vi "Climb.vi"(11 "Buttons":bool[](array[boolean])) -> ()   [LabVIEW 2015]
uses:
  Utilities/ReadyClimber.ctl
  Utilities/Climb.ctl
  Utilities/GeneralGlobals.vi
  Utilities/MotorPositionGlobals.vi
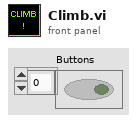
[diagram p1: front panel]
types:
  T1 = typedef "Climb.ctl" = enum16{"WaitingForInput", "ArmUp", "CloseServo", "Climb"}
  T2 = typedef "ReadyClimber.ctl" = enum16{"WaitingForInput", "ArmUp", "OpenServo", "LiftUp"}
  T3 = typedef "WPI_MotorControlDeviceRef.ctl" = cluster{"DeviceStatus":errorcluster, "Type":T4, "PWM":cluster{"PWM Channel":T5, "DeadBand":T6}, "CAN":cluster{"Device Number":u8, "Control Mode":T7, "Semaphore":T8, "Max Vout":dbl, "TalonSRX Control Mode":T9}, "Invert":bool}
  T4 = typedef "WPI_MotorControlType.ctl" = enum16{"PWM", "CAN", "CANTalonSRX"}
  T5 = typedef "FPGA_DIOPWMChannel.ctl" = enum8{"PWM 0", "PWM 1", "PWM 2", "PWM 3", "PWM 4", "PWM 5", "PWM 6", "PWM 7", "PWM 8", "PWM 9", "PWM MXP 0", "PWM MXP 1", "PWM MXP 2", "PWM MXP 3", "PWM MXP 4", "PWM MXP 5", "PWM MXP 6", "PWM MXP 7", "PWM MXP 8", "PWM MXP 9", "Invalid"}
  T6 = typedef "WPI_PWMDeadband.ctl" = cluster{"Name":string, "maxPositivePwm":i32, "minPositivePwm":i32, "centerPwm":i32, "maxNegativePwm":i32, "minNegativePwm":i32, "angularRange":u16}
  T7 = typedef "WPI_CANJaguar_ControlMode.ctl" = enum8{"Percent VBus", "Current", "Speed", "Position", "Voltage"}
  T8 = typedef "Semaphore RefNum" = refnum<k1>
  T9 = typedef "WPI_CANTalonSRX_APIControlMode.ctl" = enum8{"Percent VBus", "Speed", "Position", "Slave", "Unchanged / Invalid", "Voltage Compensation", "Current", "Motion Profile"}
  T10 = typedef "WPI_ServoDeviceRef.ctl" = cluster{"DeviceStatus":errorcluster, "PWM Channel":T5, "DeadBand":T6}
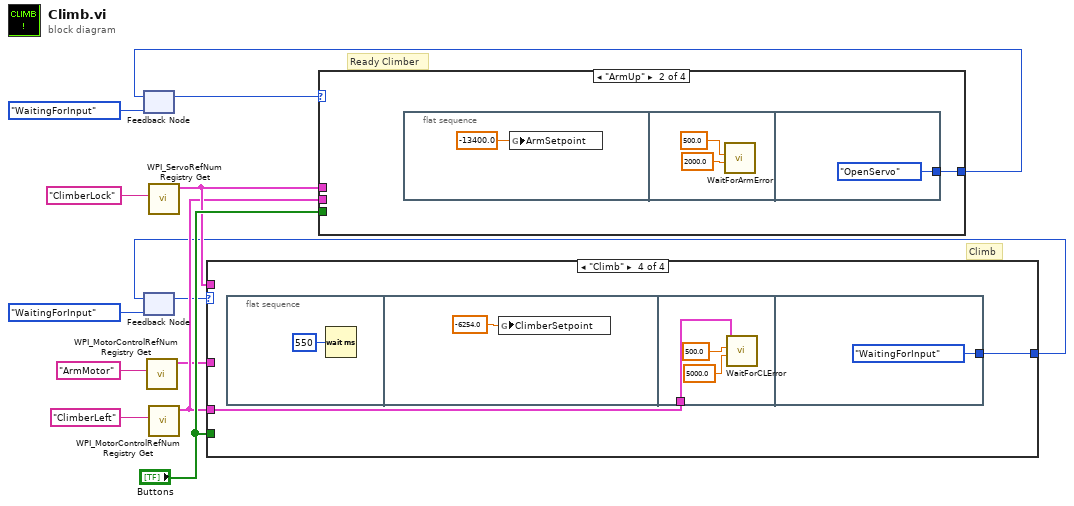
[diagram p0: block diagram]
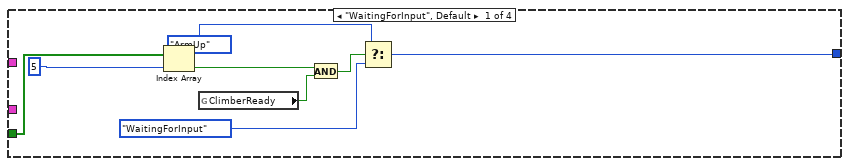
[diagram p2: hidden frame]
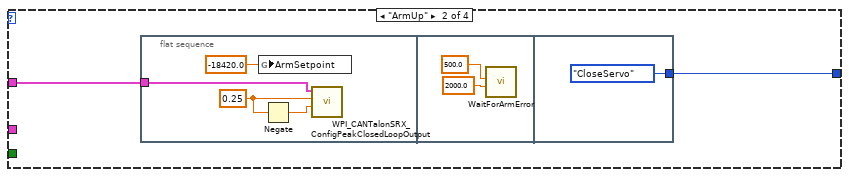
[diagram p3: hidden frame]
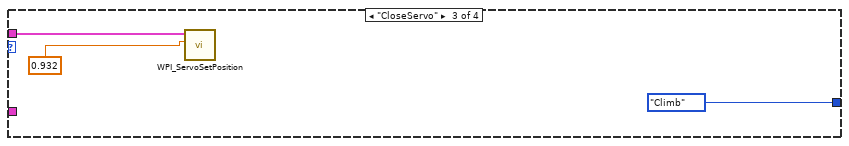
[diagram p4: hidden frame]
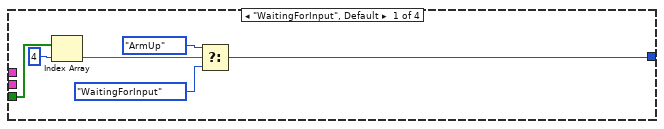
[diagram p5: hidden frame]
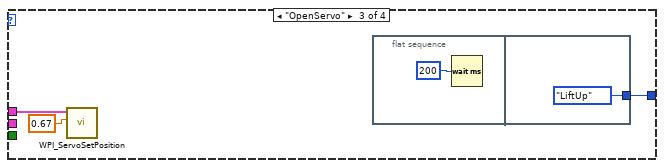
[diagram p6: hidden frame]
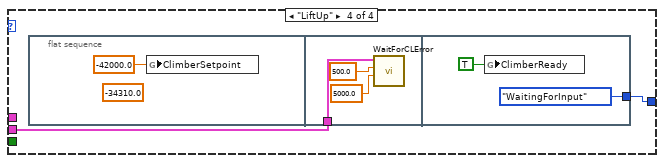
[diagram p7: hidden frame]
diagram:
  # "Climb"
  # "Ready Climber"
  n1 = feedback #1(ReadyClimber."WaitingForInput" ("Enum")) -> (w10:T2)
  n2 = feedback #2(Climb."WaitingForInput" ("Enum")) -> (w4:T1)
  n3 = call <vilib>:"WPI_MotorControlRefNum Registry Get.vi"("refnum name"="ArmMotor") -> ("MotorControlDevRef"=w1:T3)  [unwired: 9 in, 1 out]
  n4 = call <vilib>:"WPI_ServoRefNum Registry Get.vi"("refnum name"="ClimberLock") -> ("ServoDeviceRef"=w7:T10)  [unwired: 9 in, 1 out]
  n5 = call <vilib>:"WPI_MotorControlRefNum Registry Get.vi"("refnum name"="ClimberLeft") -> ("MotorControlDevRef"=w5:T3)  [unwired: 9 in, 1 out]
  n6 = case shown="\"Climb\"" w4 {
    tunnel: "Buttons" -> [w20 _ _ _]
    tunnel: w7 -> [_ _ w32 _]
    tunnel: w5 -> [_ _ _ w35]
    tunnel: [w17 w23 Climb."Climb" ("Enum") w34] -> w3
    tunnel: w1 -> [_ w22 _ _]
    frame "WaitingForInput", Default {
      n7 = Index Array(array=w20, index=5) -> (element=w16:bool)
      n8 = global read "GeneralGlobals.vi" "ClimberReady"() -> (w15:bool)
      n9 = And(x=w16, y=w15) -> (x .and. y?=w14:bool)
      n10 = Select(t=Climb."ArmUp" ("Enum"), s=w14, f=Climb."WaitingForInput" ("Enum")) -> (s? t:f=w17:T1)
    }
    frame "ArmUp" {
      n11 = flat-sequence {
        tunnel: w22 -> [w26]
        tunnel: [Climb."CloseServo" ("Enum")] -> w23
        frame #0 {
          w25 = 0.25 ("Forward Peak Output")
          n12 = global write "MotorPositionGlobals.vi" "ArmSetpoint"(-18420.0 ("ArmSetpoint")) -> ()
          n13 = Negate(x=w25) -> (-x=w24:dbl)
          n14 = call <vilib>:"WPI_CANTalonSRX_ConfigPeakClosedLoopOutput.vi"("Reverse Peak Output"=w24, "Forward Peak Output"=w25, "CAN Talon SRX Ref"=w26) -> ()  [unwired: 7 in, 2 out]
        }
        frame #1 {
          n15 = call "WaitForArmError.vi"("Timeout (ms)"=2000.0, "AllowedError"=500.0) -> ()  [unwired: 9 in, 1 out]
        }
        frame #2 {
        }
      }
    }
    frame "CloseServo" {
      n16 = call <vilib>:"WPI_ServoSetPosition.vi"("Position"=0.932, "ServoDeviceRef"=w32) -> ()  [unwired: 8 in, 2 out]
    }
    frame "Climb" {
      n17 = flat-sequence {
        tunnel: w35 -> [w40]
        tunnel: [Climb."WaitingForInput" ("Enum")] -> w34
        frame #0 {
          n18 = Wait (ms)(milliseconds to wait=u32 550) -> ()  [unwired: 1 out]
        }
        frame #1 {
          n19 = global write "MotorPositionGlobals.vi" "ClimberSetpoint"(-6254.0 ("ClimberSetpoint")) -> ()
        }
        frame #2 {
          n20 = call "WaitForCLError.vi"("Timeout (ms)"=5000.0, "AllowedError"=500.0, "CAN Talon SRX Ref"=w40) -> ()  [unwired: 8 in, 1 out]
        }
        frame #3 {
        }
      }
    }
  }
  n21 = feedback-in #2(w3) -> ()
  n22 = case shown="\"ArmUp\"" w10 {
    tunnel: "Buttons" -> [w43 _ _ _]
    tunnel: [w42 w48 w54 w58] -> w9
    tunnel: w7 -> [_ _ w55 _]
    tunnel: w5 -> [_ _ _ w59]
    frame "WaitingForInput", Default {
      n23 = Index Array(array=w43, index=4) -> (element=w46:bool)
      n24 = Select(t=ReadyClimber."ArmUp" ("Enum"), s=w46, f=ReadyClimber."WaitingForInput" ("Enum")) -> (s? t:f=w42:T2)
    }
    frame "ArmUp" {
      n25 = flat-sequence {
        tunnel: [ReadyClimber."OpenServo" ("Enum")] -> w48
        frame #0 {
          n26 = global write "MotorPositionGlobals.vi" "ArmSetpoint"(-13400.0 ("ArmSetpoint")) -> ()
        }
        frame #1 {
          n27 = call "WaitForArmError.vi"("Timeout (ms)"=2000.0, "AllowedError"=500.0) -> ()  [unwired: 9 in, 1 out]
        }
        frame #2 {
        }
      }
    }
    frame "OpenServo" {
      n28 = call <vilib>:"WPI_ServoSetPosition.vi"("Position"=0.67, "ServoDeviceRef"=w55) -> ()  [unwired: 8 in, 2 out]
      n29 = flat-sequence {
        tunnel: [ReadyClimber."LiftUp" ("Enum")] -> w54
        frame #0 {
          n30 = Wait (ms)(milliseconds to wait=u32 200) -> ()  [unwired: 1 out]
        }
        frame #1 {
        }
      }
    }
    frame "LiftUp" {
      n31 = flat-sequence {
        tunnel: w59 -> [w63]
        tunnel: [ReadyClimber."WaitingForInput" ("Enum")] -> w58
        frame #0 {
          (unwired) -34310.0 ("ClimberSetpoint")
          n32 = global write "MotorPositionGlobals.vi" "ClimberSetpoint"(-42000.0 ("ClimberSetpoint")) -> ()
        }
        frame #1 {
          n33 = call "WaitForCLError.vi"("Timeout (ms)"=5000.0, "AllowedError"=500.0, "CAN Talon SRX Ref"=w63) -> ()  [unwired: 8 in, 1 out]
        }
        frame #2 {
          n34 = global write "GeneralGlobals.vi" "ClimberReady"(TRUE ("ClimberReady")) -> ()
        }
      }
    }
  }
  n35 = feedback-in #1(w9) -> ()
